vi "Colour wave.vi"(11 "Numeric":i32) -> (3 "Array":u32[](array[numeric]))   [LabVIEW 2025]
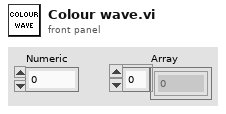
[diagram p1: front panel]
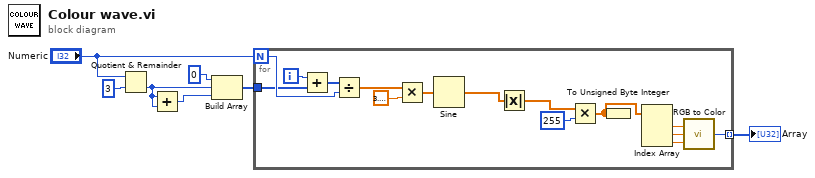
[diagram p0: block diagram]
diagram:
  n1 = Quotient & Remainder(x="Numeric", y=3) -> (floor(x/y)=w4:i32)  [unwired: 1 out]
  n2 = Add(x=w4, y=w4) -> (x+y=w5:i32)
  n3 = Build Array(0, w4, w5) -> (w6:i32[])
  n4 = for {
    N: "Numeric" -> [w21]
    tunnel: w6 -> [w16]
    tunnel: [w13] -> w7 mode=indexing
    i -> [w22]
    n5 = Add(x=w22, y=w16) -> (x+y=w17:i32[])
    n6 = Divide(x=w17, y=w21) -> (x/y=w20:dbl[])
    n7 = Multiply(x=w20, y=3.141592653589793) -> (x*y=w18:dbl[])
    n8 = Sine(x=w18) -> (sin(x)=w12:dbl[])
    n9 = Absolute Value(x=w12) -> (abs(x)=w15:dbl[])
    n10 = Multiply(x=w15, y=255) -> (x*y=w11:dbl[])
    n11 = To Unsigned Byte Integer(number=w11) -> ()  [unwired: 1 out]
    n12 = Index Array(array=w11) -> (element #1=w10:dbl, element #2=w9:dbl, element #3=w8:dbl)  [unwired: 3 in]
    n13 = call <vilib>:"RGB to Color.vi"("B"=w8, "G"=w9, "R"=w10) -> ("Color"=w13:u32)
  }
  "Array" <- w7
